vi "position_adj.vi"(1 "coordinate.y":i16, 2 "coordinate.x":i16, 3 "image data in":T1) -> (0 "image data out":T1)   [LabVIEW 2018]
uses:
  <vilib>/picture/picture.llb/imagedata.ctl
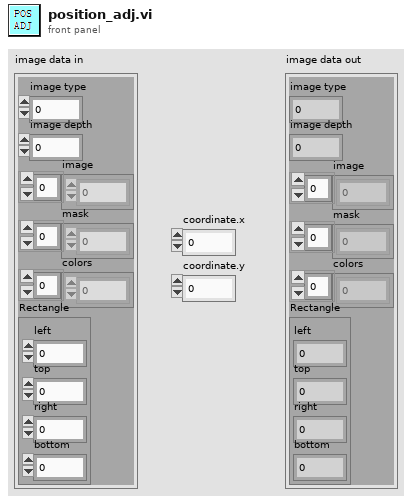
[diagram p1: front panel]
types:
  T1 = typedef "imagedata.ctl" = cluster{"image type":i32, "image depth":i32, "image":u8[], "mask":u8[], "colors":u32[], "Rectangle":cluster{"left":i16, "top":i16, "right":i16, "bottom":i16}}
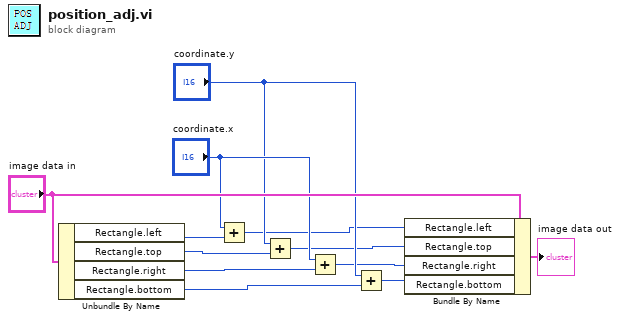
[diagram p0: block diagram]
diagram:
  n1 = Unbundle By Name("image data in") -> ("Rectangle.left"=w9:i16, "Rectangle.top"=w10:i16, "Rectangle.right"=w8:i16, "Rectangle.bottom"=w7:i16)
  n2 = Add(x="coordinate.x", y=w9) -> (x+y=w4:i16)
  n3 = Add(x="coordinate.y", y=w10) -> (x+y=w3:i16)
  n4 = Add(x="coordinate.x", y=w8) -> (x+y=w2:i16)
  n5 = Add(x="coordinate.y", y=w7) -> (x+y=w1:i16)
  n6 = Bundle By Name(cluster="image data in", "Rectangle.left"=w4, "Rectangle.top"=w3, "Rectangle.right"=w2, "Rectangle.bottom"=w1) -> (→"image data out":T1)
